vi "initAcq.vi"(8 "error in (no error)":errorcluster, 11 "Acquisition in":refnum<class "Acquisition.lvclass">) -> (0 "error out":errorcluster, 3 "Acquisition out":refnum<class "Acquisition.lvclass">)   [LabVIEW 2014, in "Acquisition.lvclass"]
uses:
  Acquisition.lvclass
  Database/Database.lvclass
  Acquisition.lvclass/Acquisition.ctl
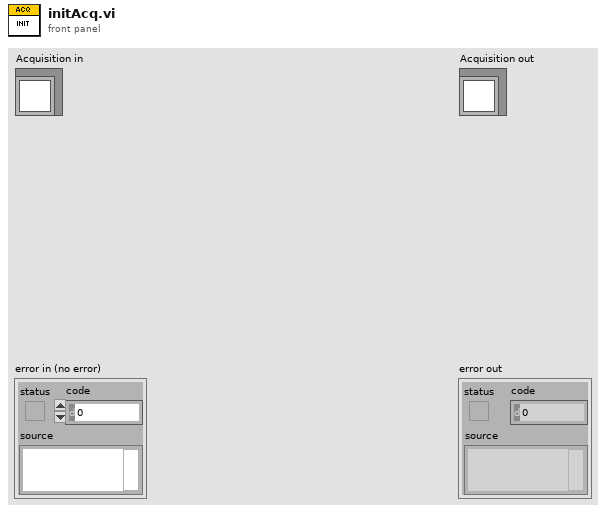
[diagram p1: front panel]
types:
  T1 = cluster{"timestamp":dbl, "stimulus":string, "trial":dbl}
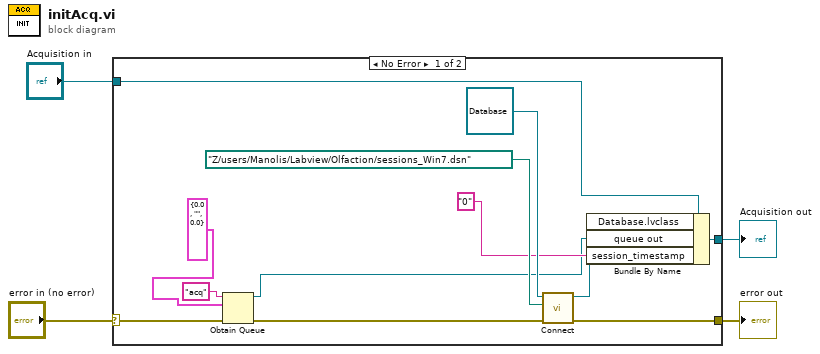
[diagram p0: block diagram]
diagram:
  n1 = case shown="No Error" "error in (no error)" {
    selector: "error in (no error)" -> [w9 w18]
    tunnel: [w15 w18] -> w3
    tunnel: [w13 w17] -> w1
    tunnel: "Acquisition in" -> [w14 w17]
    frame No Error {
      n2 = Obtain Queue(name (unnamed)="acq", element data type=T1 {"timestamp"=0.0, "stimulus"="", "trial"=0.0} ("element"), error in (no error)=w9) -> (queue out=w5:refnum<queue>, error out=w8:errorcluster)  [unwired: 2 in, 1 out]
      n3 = call-dynamic "Connect.vi"("error in (no error)"=w8, "Session"=path "Z:/users/Manolis/Labview/Olfaction/sessions_Win7.dsn", "Database in"=refnum<class "Database.lvclass"> refnum ("Database.lvclass")) -> ("error out"=w15:errorcluster, "Database out"=w12:refnum<class "Database.lvclass">)  [unwired: 7 in]
      n4 = Bundle By Name(cluster=w14, "Database.lvclass"=w12, "queue out"=w5, "session_timestamp"="0") -> (w13:refnum<class "Acquisition.lvclass">)
    }
    frame Error {
    }
  }
  "error out" <- w3
  "Acquisition out" <- w1
